vi "Save Encoder Data From MyRio_sub_VI.vi"() -> (3 "Output String":string)   [LabVIEW 2017]
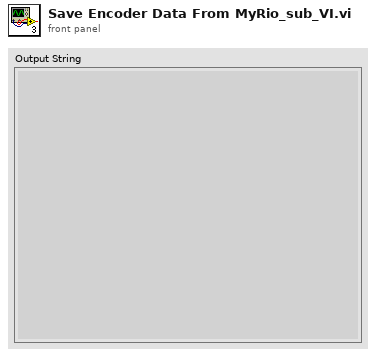
[diagram p1: front panel]
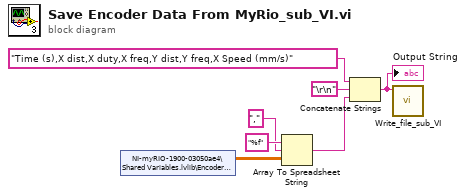
[diagram p0: block diagram]
diagram:
  n1 = shared-variable "NI-myRIO-1900-03050ae4\\Shared Variables.lvlib\\Encoder Data"() -> (w7:dbl[][])  [unwired: 1 in, 1 out]
  n2 = Array To Spreadsheet String(delimiter (Tab)=",", array=w7, 3:"%f" ("format string")) -> (spreadsheet string=w6:string)
  n3 = Concatenate Strings("Time (s),X dist,X duty,X freq,Y dist,Y freq,X Speed (mm/s)", "\r\n", w6) -> (w5:string)
  "Output String" <- w5
  n4 = call "Write_file_sub_VI.vi"("Output String"=w5) -> ()  [unwired: 9 in, 2 out]
